vi "Switch.vi"(7 "Use Ch0":bool, 8 "Ch1 Q":fxp<+/-,32,14>, 9 "Ch1 I":fxp<+/-,32,14>, 10 "Ch0 Q":fxp<+/-,32,14>, 11 "Ch0 I":fxp<+/-,32,14>) -> (2 "Out Q":fxp<+/-,32,14>, 3 "Out I":fxp<+/-,32,14>)   [LabVIEW 2018]
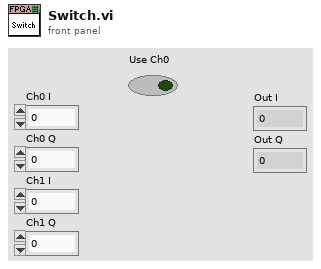
[diagram p1: front panel]
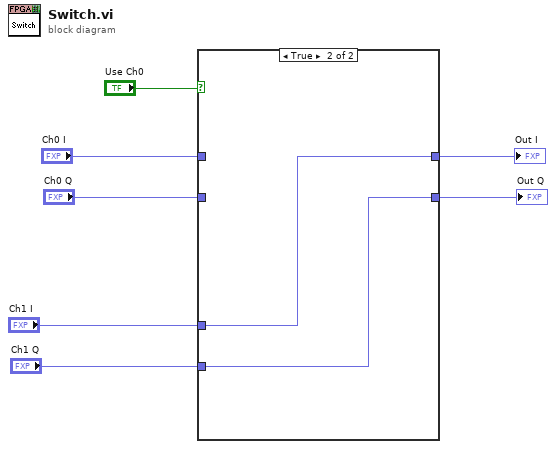
[diagram p0: block diagram]
diagram:
  n1 = case shown="True" "Use Ch0" {
    tunnel: [w9 w11] -> w6
    tunnel: "Ch0 I" -> [w9 _]
    tunnel: [w8 w10] -> w4
    tunnel: "Ch0 Q" -> [w8 _]
    tunnel: "Ch1 I" -> [_ w11]
    tunnel: "Ch1 Q" -> [_ w10]
    frame False {
    }
    frame True {
    }
  }
  "Out I" <- w6
  "Out Q" <- w4
